vi "Save FIR coeff to CSV.vi"(8 "error in (no error)":T1, 10 "EQ FIR coeff":cdb[](array[numeric]), 11 "Path":path) -> (0 "error out":T1)   [LabVIEW 2019]
uses:
  <vilib>/Utility/file.llb/Write Delimited Spreadsheet (string).vi
  <vilib>/Utility/file.llb/Write Delimited Spreadsheet (DBL).vi
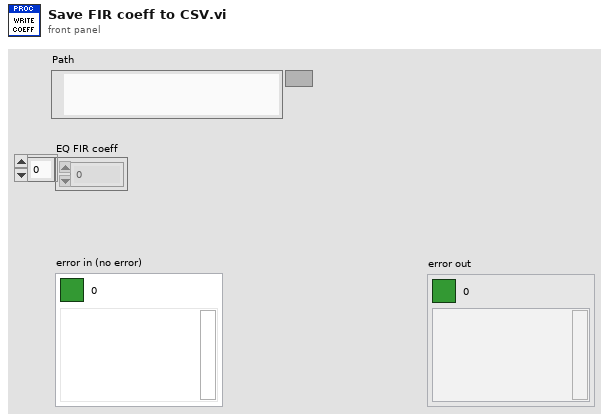
[diagram p1: front panel]
types:
  T1 = cluster{"Boolean Round":bool, "code":i32, "source":string}
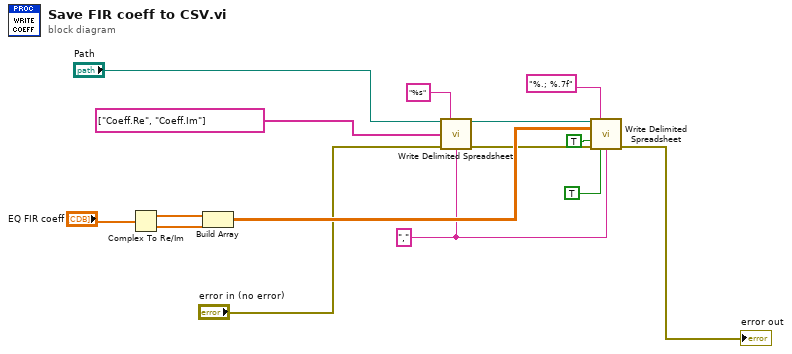
[diagram p0: block diagram]
diagram:
  w1 = "," ("delimiter (\\t)")
  n1 = Complex To Re/Im(x + iy="EQ FIR coeff") -> (x=w14:dbl[], y=w13:dbl[])
  n2 = Build Array(w14, w13) -> (w7:dbl[][])
  n3 = call-poly <vilib>:"Write Delimited Spreadsheet.vi"("file path (dialog if empty)"="Path", "format (%s)"="%s" ("format (%.3f)"), "1D data"=string[] ["Coeff.Re", "Coeff.Im"] ("format (%.3f)"), "error in (no error)"="error in (no error)", "delimiter (\\t)"=w1) -> ("new file path (Not A Path if cancelled)"=w8:path, "error out"=w3:errorcluster)  [unwired: 9 in]
  n4 = call-poly <vilib>:"Write Delimited Spreadsheet.vi"("file path (dialog if empty)"=w8, "format (%.3f)"="%.; %.7f" ("format string"), "2D data"=w7, "append to file? (new file:F)"=TRUE, "error in (no error)"=w3, "transpose? (no:F)"=TRUE, "delimiter (\\t)"=w1) -> ("error out"=→"error out":errorcluster)  [unwired: 7 in, 1 out]
